vi "Set Time.vi"(8 "error in (no error)":errorcluster, 10 "Time":T1, 11 "Device ID (0)":i32) -> (0 "error out":errorcluster, 3 "Device ID out":i32)   [LabVIEW 8.6, in "Keyence LJ-V7000.lvlib"]
doc: "This function sets the date/time for the controller."
uses:
  Keyence LJ-V7000.lvlib
  constant/Driver VI No.ctl
  Clusters/Time.ctl
panel:
  # "(c) 2012 KEYENCE CORPORATION.  ALL RIGHTS RESERVED."
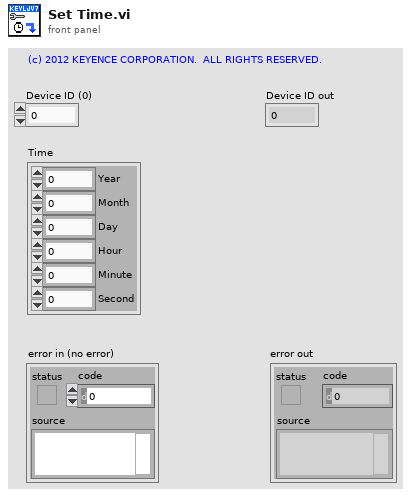
[diagram p1: front panel]
types:
  T1 = typedef "Keyence LJ-V7000.lvlib/Time.ctl" = cluster{"Year":u8, "Month":u8, "Day":u8, "Hour":u8, "Minute":u8, "Second":u8}
  T2 = typedef "Keyence LJ-V7000.lvlib/Driver VI No.ctl" = enum16{"Initialize", "Close", "Reboot Controller", "Return to Factory State", "Get System Error", "Clear System Error", "Trigger", "Start Batch Measurements", "Stop Batch Measurements", "Auto Zero", "Timing", "Reset", "Clear Memory", "Set Setting", "Get Setting", "Initialize Setting", "Reflect Setting", "Update Write Settings Area", "Check Status of Saving to Save Area", "Set Time", "Get Time", "Change Program", "Read Active Program Number", "Read Measurement Data", "Read Profiles(for High-Speed Mode)", "Read Batch Profiles(for High-Speed Mode)", "Read Profiles(for Advanced Mode)", "Read Batch Profiles(for Advanced Mode)", "Start Storage", "Stop Storage", "Read Storage Status", "Read Data Storage Data", "Read Profile Storage Data", "Read Batch Profile Storage Data", "Start High-Speed Data Communication", "Stop High-Speed Data Communication", "Read Profiles(for High-Speed Communication)"}
  T3 = cluster{"Year":u8, "Month":u8, "Day":u8, "Hour":u8, "Minute":u8, "Second":u8, "reserve":u8, "reserve":u8}
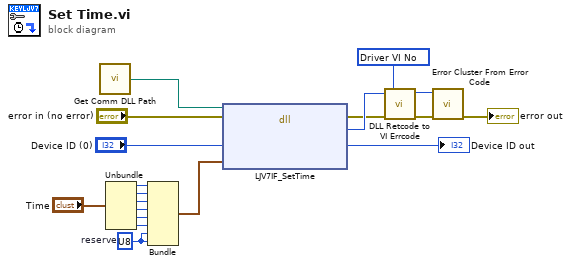
[diagram p0: block diagram]
diagram:
  w8 = u8 ?  # reserve
  n1 = call "Get Comm DLL Path.vi"() -> ("Comm DLL Path"=w17:path)  [unwired: 1 in]
  n2 = Unbundle("Time") -> ("Year"=w14:u8, "Month"=w13:u8, "Day"=w12:u8, "Hour"=w11:u8, "Minute"=w10:u8, "Second"=w9:u8)
  n3 = Bundle("Year"=w14, "Month"=w13, "Day"=w12, "Hour"=w11, "Minute"=w10, "Second"=w9, "reserve"=w8, "reserve"=w8) -> (w7:T3)  [unwired: 1 in]
  n4 = dll-call lib="C:/Program Files/National Instruments/LabVIEW 2011/instr.lib/Keyence LJ-V7000/LJV7_IF.*" fn="LJV7IF_SetTime"(path in=w17, error in="error in (no error)", "lDeviceId"="Device ID (0)", "pTime"=w7) -> (error out=w3:errorcluster, "lRetCode"=w4:i32, "lDeviceId"=→"Device ID out":i32)  [unwired: 2 in, 1 out]
  n5 = call "DLL Retcode to VI Errcode.vi"("Driver VI No"=T2 ?, "error in (no error)"=w3, "DLL Return Code"=w4) -> ("error out"=w6:errorcluster, "VI Error Code"=w5:i32)  [unwired: 7 in]
  n6 = call <vilib>:"Error Cluster From Error Code.vi"("error in (no error)"=w6, "error code (0)"=w5) -> ("error out"=→"error out":errorcluster)  [unwired: 7 in]
